vi "EMC_VEL_Move.vi"(8 "error in (no error)":errorcluster, 10 "Motion Parameters":T1={"position"=1000.0, "velocity"=1000.0, "acceleration"=10000.0, "deceleration"=10000.0, "accel. jerk"=10000.0, "decel. jerk"=10000.0}, 11 "axis":refnum<k21>) -> (0 "error out":errorcluster)   [LabVIEW 2015]
uses:
  EMC_Typedef_Motor_Parameters.ctl
  <vilib>/Motion/PropertyNodes/nimc.createStraightLineMoveInstance.axis.vi
  <vilib>/Motion/PropertyNodes/nimc.destroyInterfaceInstance.vi
  <resource>/objmgr/nimotion.rc
panel:
  out "Numeric":i32
  in  "table":refnum<k21>
  in  "coordinate":refnum<k21>
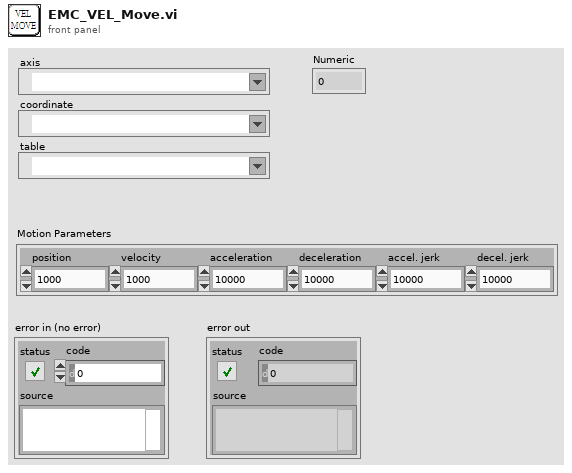
[diagram p1: front panel]
types:
  T1 = typedef "EMC_Typedef_Motor_Parameters.ctl" = cluster{"position":dbl, "velocity":dbl, "acceleration":dbl, "deceleration":dbl, "accel. jerk":dbl, "decel. jerk":dbl}
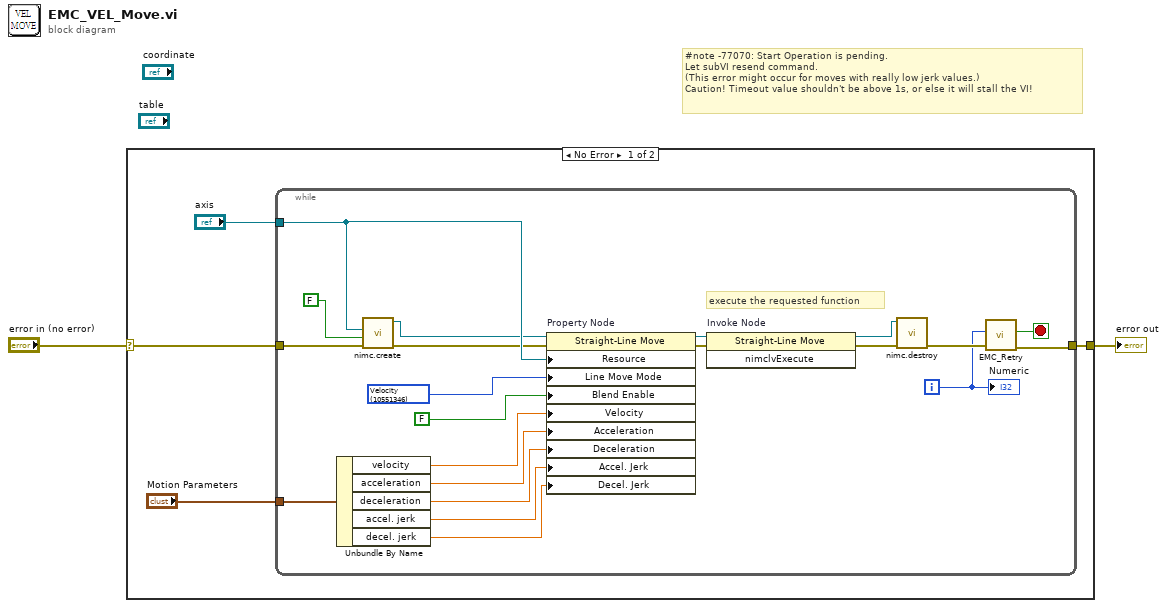
[diagram p0: block diagram]
diagram:
  # "#note -77070: Start Operation is pending.\nLet subVI resend command.\n(This error might occur for moves with really low jerk values.)\nCaution! Timeout value shouldn't be above 1s, or else it will stall the VI!"
  n1 = case shown="No Error" "error in (no error)" {
    selector: "error in (no error)" -> [w3 w28]
    tunnel: [w6 w28] -> w2
    frame No Error {
      n2 = while {
        tunnel: [w9] -> w6
        tunnel: "Motion Parameters" -> [w21]
        tunnel: "axis" -> [w14]
        tunnel: w3 -> [w13]
        i -> [w7]
        stop <- w8 stop-if-true
        w15 = 10551346 items=["Relative"=10551344, "Absolute"=10551337, "Relative To Capture"=10551345, "Velocity"=10551346, "Polyline"=11600101] ("line move mode")
        # "execute the requested function"
        n3 = Unbundle By Name(w21) -> ("velocity"=w20:dbl, "acceleration"=w19:dbl, "deceleration"=w18:dbl, "accel. jerk"=w17:dbl, "decel. jerk"=w16:dbl)
        n4 = call-poly <vilib>:"nimc.create.vi"("error in"=w13, "async?"=FALSE ("execute asynchronously?"), "axis"=w14) -> ("error out"=w11:errorcluster, "line"=w12:refnum<k20>)  [unwired: 6 in, 1 out]
        n5 = property on="Property Node" class="Straight-Line Move"(reference=w12, error in=w11, "Resource"=w14, "Line Move Mode"=w15, "Blend Enable"=FALSE ("blend enable"), "Velocity"=w20, "Acceleration"=w19, "Deceleration"=w18, "Accel. Jerk"=w17, "Decel. Jerk"=w16) -> (reference out=w27:refnum<k20>, error out=w26:errorcluster)
        n6 = invoke on="Invoke Node" class="Straight-Line Move" method="nimclvExecute"(reference=w27, error in=w26) -> (reference out=w24:refnum<k20>, error out=w23:errorcluster)  [unwired: 1 in, 1 out]
        n7 = call-poly <vilib>:"nimc.destroy.vi"("error in"=w23, "motion handle"=w24) -> ("error out"=w10:errorcluster)  [unwired: 9 in]
        n8 = call "EMC_Retry.vi"("error in (no error)"=w10, "Count in"=w7) -> ("error out"=w9:errorcluster, "Exit"=w8:bool)  [unwired: 8 in]
        "Numeric" <- w7
      }
    }
    frame Error {
    }
  }
  "error out" <- w2
